vi "Wavelet Packet - Read Entropy.vi"() -> ()   [LabVIEW 2023]
doc: "This example shows how to read the wavelet packet coefficients and the corresponding entropy value of a certain node with the WA WP Read Node and the WA WP Read Entropy VI, respectively.\n\n<b>Instructions:</b>\n1) Run this VI.\n2) Observe the <b>Node Coefficients</b> and the <b>Entropy</b>.\n3) Change the value of <b>Path</b> to obtain the coefficients at other nodes.\n4) Browse the Block Diagram to learn how to read coefficients and entropy from a wavelet packet tree."
uses:
  <vilib>/addons/Wavelet Analysis/wavelet packet.llb/WA WP Decomposition (Waveform).vi
  <vilib>/addons/_Advanced Signal Processing/NI_AdvSigProcWA.lvlib
panel:
  in  "Data":u16(ring)=115 items=["1D Example Data"=100, "-"=101, "Doppler"=102, "HOP"=103, "TF Sine"=104, "Noisy Doppler"=105, "Sea Temperature"=106, "Sp500"=107, "Power Line"=108, "Engine Knocking"=109, "HeaviSine"=110, "Bumps"=111, "Blocks"=112, "Piece Regular"=113, "HypChirps"=114, "LinChirps"=115, "Chirps"=116, "Piece Polynomial"=117, "ECG"=131, "-"=118, "2D Example Data"=119, "-"=120, "Finger Print (Image)"=121, "Iris Flower (Image)"=122, "Mammogram (Image)"=123, "Lake (Image)"=127, "Two Can 1 (Image)"=132, "Two Can 2 (Image)"=133, "Camera Man (Image)"=134]
  out "Signal":waveform(dbl)(graph)
  out "Entropy":dbl format="%.2f"
  out "Node Coefficients":dbl[](graph)
  in  "Path":string="0001"
  in  "Wavelet":u16(ring) items=["db02"=0, "db03"=1, "db04"=2, "db05"=3, "db06"=4, "db07"=5, "db08"=6, "db09"=7, "db10"=8, "db11"=9, "db12"=10, "db13"=11, "db14"=12, "Haar"=13, "bior1_3"=14, "bior1_5"=15, "bior2_2"=16, "bior2_4"=17, "bior2_6"=18, "bior2_8"=19, "bior3_1"=20, "bior3_3"=21, "bior3_5"=22, "bior3_7"=23, "bior3_9"=24, "bior4_4 (FBI)"=25, "bior5_5"=38, "bior6_8"=39, "coif1"=26, "coif2"=27, "coif3"=28, "coif4"=29, "coif5"=30, "sym2"=31, "sym3"=32, "sym4"=33, "sym5"=34, "sym6"=35, "sym7"=36, "sym8"=37]
  # "Overview: Shows how to read the wavelet packet coefficients and the corresponding entropy value of a certain node with the WA WP Read Node and the WA WP Read Entropy VI, respectively.\nRequirements: LabVIEW Full Development System, Advanced Signal Processing Toolkit\nInstructions: \n1. Run this VI.\n2. Observe the Node Coefficients and the Entropy.\n3. Change the value of Path to obtain the coefficients at other nodes.\n4. Browse the block diagram to learn how to read coefficients and entropy from a wavelet packet tree."
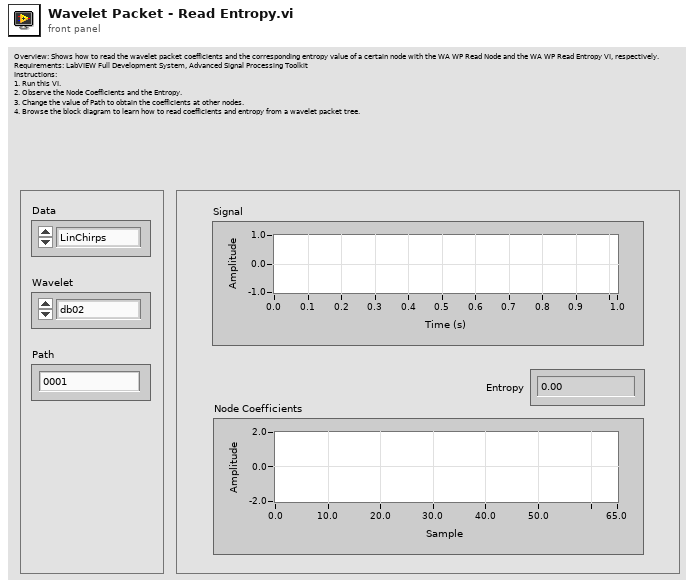
[diagram p1: front panel]
types:
  T1 = typedef "NI_AdvSigProcWA.lvlib/WA Generic Ref.ctl" = cluster{"ref":u64, "t0":timestamp, "dt":dbl}
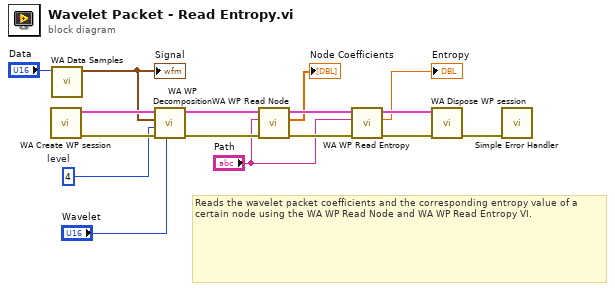
[diagram p0: block diagram]
diagram:
  w10 = 4  # level
  # "Reads the wavelet packet coefficients and the corresponding entropy value of a certain node using the WA WP Read Node and WA WP Read Entropy VI."
  n1 = call <vilib>:"WA Create WP session.vi"() -> ("error out"=w15:errorcluster, "WP session out"=w16:T1)  [unwired: 1 in, 9 out]
  n2 = call <vilib>:"WA Data Samples.vi"("data"="Data") -> ("signal"=w4:waveform(dbl))  [unwired: 10 out]
  "Signal" <- w4
  n3 = call-poly <vilib>:"WA WP Decomposition.vi"("wavelet"="Wavelet", "error in (no error)"=w15, "levels"=w10, "signal"=w4, "WP session"=w16) -> ("error out"=w6:errorcluster, "WP session out"=w5:T1)  [unwired: 5 out]
  n4 = call <vilib>:"WA WP Read Node.vi"("error in (no error)"=w6, "path"="Path", "WP session"=w5) -> ("error out"=w13:errorcluster, "node coef"=→"Node Coefficients":dbl[], "WP session out"=w14:T1)  [unwired: 1 in, 5 out]
  n5 = call <vilib>:"WA WP Read Entropy.vi"("error in (no error)"=w13, "path"="Path", "WP session"=w14) -> ("error out"=w11:errorcluster, "entropy"=→"Entropy":dbl, "WP session out"=w12:T1)  [unwired: 1 in, 5 out]
  n6 = call <vilib>:"WA Dispose WP session.vi"("error in (no error)"=w11, "WP session"=w12) -> ("error out"=w3:errorcluster)  [unwired: 9 out]
  n7 = call <vilib>:"Simple Error Handler.vi"("error in (no error)"=w3) -> ()  [unwired: 1 in, 8 out]
